vi "Measure Statistics (Multiple).vi"(6 "Measurements":T2[](array[typedef]), 8 "error in (no error)":errorcluster, 9 "No. Reads":i32, 10 "Channels":T3, 11 "Oscilloscope in":refnum<class "Oscilloscope.lvclass">) -> (0 "error out":errorcluster, 2 "Multiple Statistics":T1(array[cluster]), 3 "Oscilloscope out":refnum<class "Oscilloscope.lvclass">)   [LabVIEW 2018, in "Oscilloscope.lvlib" / "Oscilloscope.lvclass"]
uses:
  Oscilloscope.lvclass
  Custom Controls/Analog Channels.ctl
  Custom Controls/Measurement.ctl
  Oscilloscope.lvlib
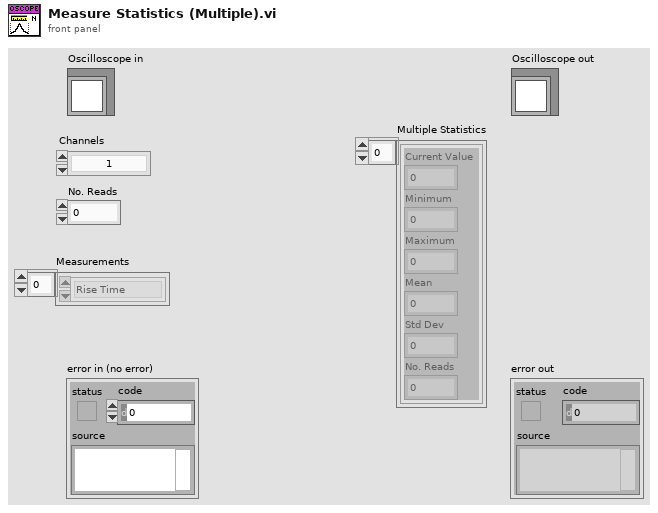
[diagram p1: front panel]
types:
  T1 = cluster{"Current Value":dbl, "Minimum":dbl, "Maximum":dbl, "Mean":dbl, "Std Dev":dbl, "No. Reads":dbl}[]
  T2 = typedef "Oscilloscope.lvlib/Measurement.ctl" = enum16{"Rise Time", "Fall Time", "Frequency", "Period", "RMS (V)", "Peak-Peak (V)", "Max (V)", "Min (V)", "High State (V)", "Low State (V)", "Average (V)", "Width (Negative)", "Width (Positive)", "Duty Cycle (Negative)", "Duty Cycle (Positive)", "Amplitude", "Cycle RMS (V)", "Cycle Avg (V)", "Overshoot", "Preshoot", "Time at Max", "Frequency Counter", "Time at Min", "Delay", "Value at Time", "Phase", "Time at Value", "Time of Edge", "Area", "Burst Width", "Falling Edge Count", "Rising Edge Count", "Falling Pulse Count", "Rising Pulse Count", "Std Dev", "Pulse Width"}
  T3 = typedef "Oscilloscope.lvlib/Analog Channels.ctl" = enum16{"1", "2", "3", "4", "5", "6", "7", "8", "9", "10", "11", "12", "13", "14", "15", "16"}
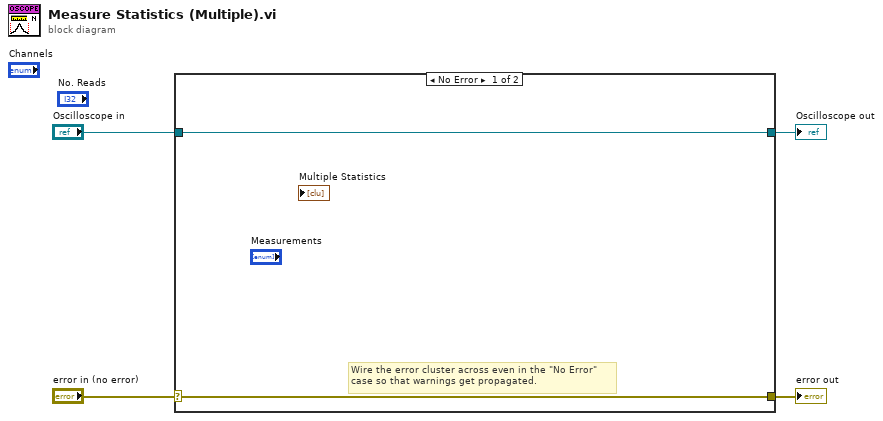
[diagram p0: block diagram]
diagram:
  n1 = case shown="No Error" "error in (no error)" {
    selector: "error in (no error)" -> [w5 w8]
    tunnel: [w5 w8] -> w3
    tunnel: [w6 w7] -> w1
    tunnel: "Oscilloscope in" -> [w6 w7]
    frame No Error {
      # "Wire the error cluster across even in the \"No Error\"\ncase so that warnings get propagated."
    }
    frame Error {
    }
  }
  "error out" <- w3
  "Oscilloscope out" <- w1
